vi "GetInstalledVIPMPackages.vi"(7 "labview version":string, 8 "error in":errorcluster) -> (0 "error out":errorcluster, 3 "array":string[](array[string]))   [LabVIEW 2019]
uses:
  <vilib>/JKI/VIPM API/VIPM API_vipm_api.lvlib
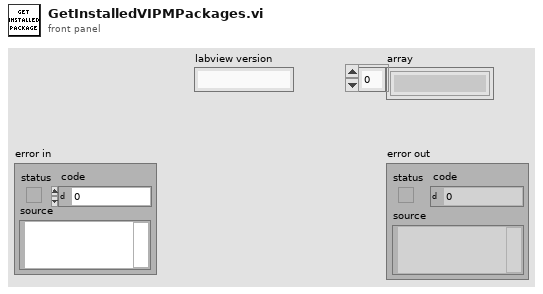
[diagram p1: front panel]
types:
  T1 = typedef "VIPM API_vipm_api.lvlib/Library Contents Cluster_vipm_api.ctl" = cluster{"Package Name":string, "Version":string, "Display Name":string, "Repository Name":string, "Company Name":string, "License Type":string, "Installed":bool, "Deprecated":bool, "Dependency or Conflict Problem":bool, "Downloaded":bool}
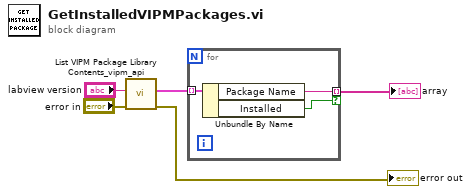
[diagram p0: block diagram]
diagram:
  n1 = call <vilib>:"List VIPM Package Library Contents_vipm_api.vi"("error in (no error)"="error in", "LabVIEW Version"="labview version") -> ("error out"=→"error out":errorcluster, "Library Contents []"=w4:T1[])  [unwired: 7 in, 1 out]
  n2 = for {
    tunnel: w4 -> [w8] mode=indexing
    tunnel: [w7] -> w3 mode=indexing if=w6
    n3 = Unbundle By Name(w8) -> ("Package Name"=w7:string, "Installed"=w6:bool)
  }
  "array" <- w3
